vi "Inicializar.vi"() -> ()   [LabVIEW 2020]
panel:
  in  "stop":bool
  out "Indicador Nombre":string
  out "Indicador Contraseña":string
  in  "Contraseña":string
  in  "Nombre":string
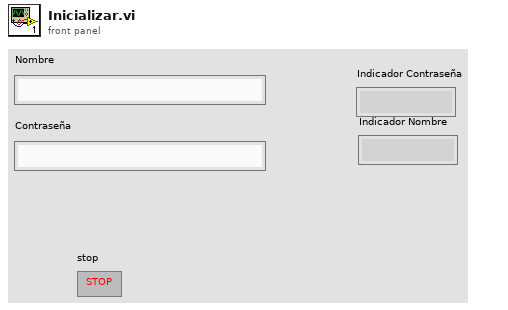
[diagram p1: front panel]
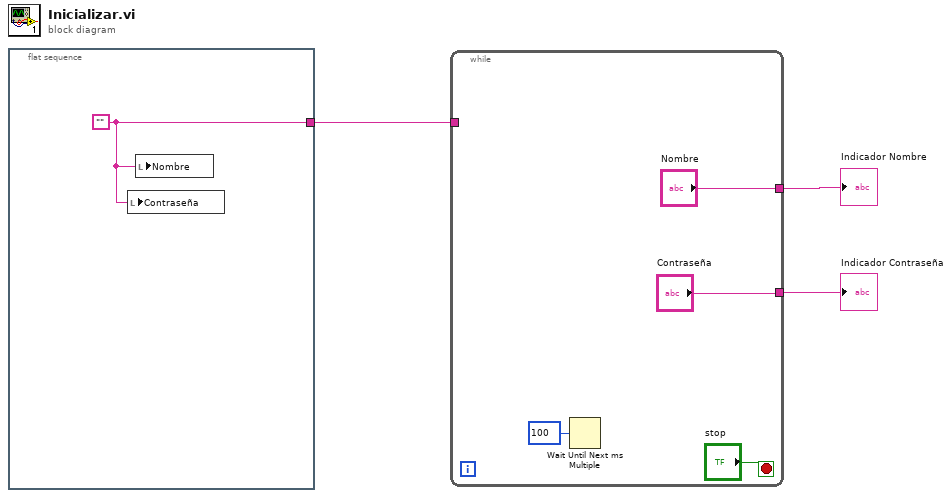
[diagram p0: block diagram]
diagram:
  n1 = flat-sequence {
    tunnel: [w4] -> w1
    frame #0 {
      w4 = ""
      n2 = local write "Contraseña"(w4) -> ()
      n3 = local write "Nombre"(w4) -> ()
    }
  }
  n4 = while {
    tunnel: ["Nombre"] -> w2
    tunnel: ["Contraseña"] -> w3
    tunnel: w1 -> [_]
    stop <- "stop" stop-if-true
    n5 = Wait Until Next ms Multiple(millisecond multiple=u32 100) -> ()  [unwired: 1 out]
  }
  "Indicador Contraseña" <- w3
  "Indicador Nombre" <- w2
